vi "Read CSV File.vi"(8 "error in (no error)":errorcluster, 11 "Serie File Name":string) -> (0 "error out":errorcluster, 3 "Serie":u16[](array[numeric]))   [LabVIEW 2018]
uses:
  <vilib>/Utility/file.llb/Read Delimited Spreadsheet (I64).vi
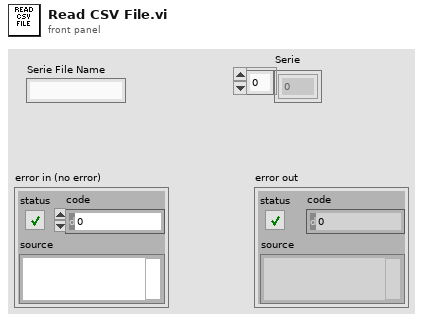
[diagram p1: front panel]
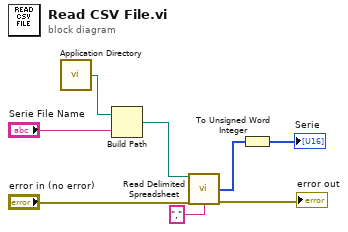
[diagram p0: block diagram]
diagram:
  n1 = call <vilib>:"Application Directory.vi"() -> ("Application Directory"=w8:path)
  n2 = Build Path(base path=w8, name or relative path="Serie File Name") -> (appended path=w6:path)
  n3 = call-poly <vilib>:"Read Delimited Spreadsheet.vi"("file path (dialog if empty)"=w6, "error in (no error)"="error in (no error)", "delimiter (\\t)"="," ("delimiter (\\t)")) -> ("first row"=w3:i64[], "error out"=→"error out":errorcluster)  [unwired: 7 in, 4 out]
  n4 = To Unsigned Word Integer(number=w3) -> (unsigned 16bit integer=→"Serie":u16[])
